vi "ModeMgr.Password Prompt.vi"(9 "Password In":string, 11 "Selected Mode":string) -> (3 "Accepted":bool)   [LabVIEW 2018]
panel:
  in  "Cancel":bool
  out "Action":string
  in  "Password":string
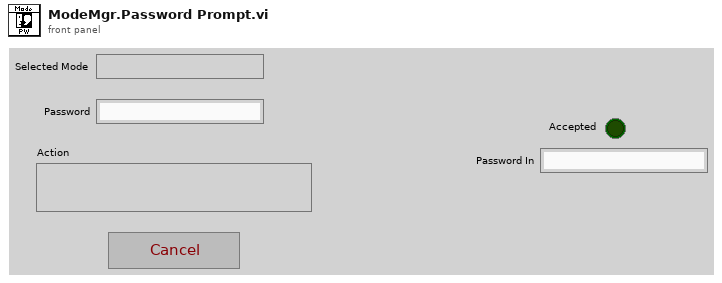
[diagram p1: front panel]
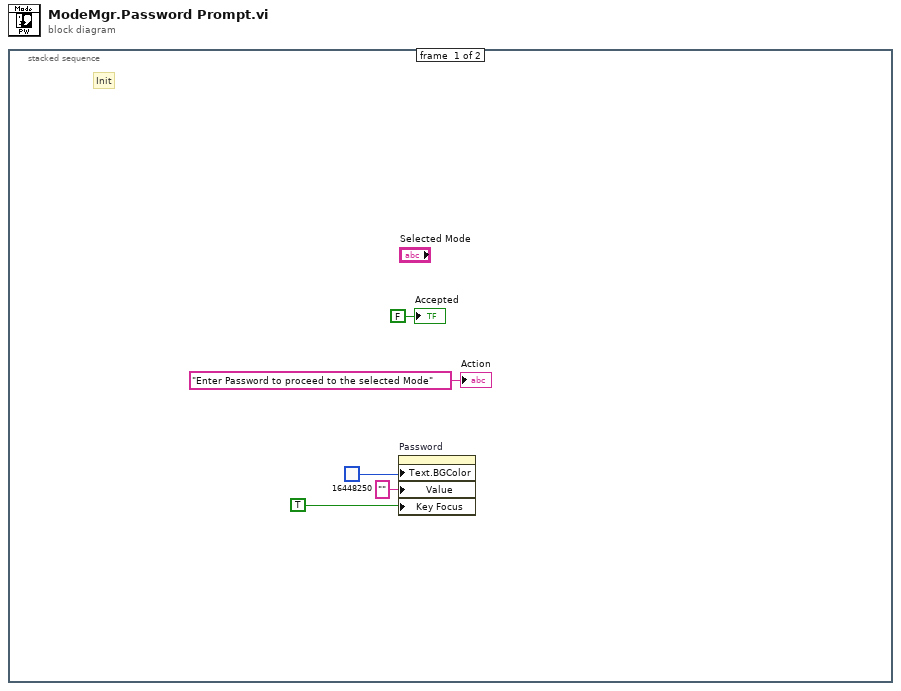
[diagram p0: block diagram]
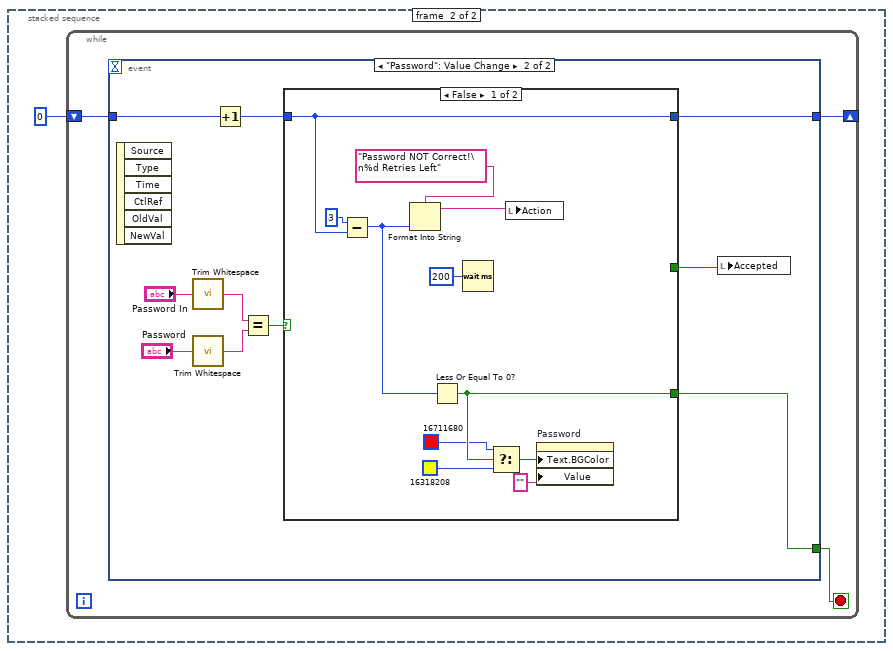
[diagram p2: hidden frame]
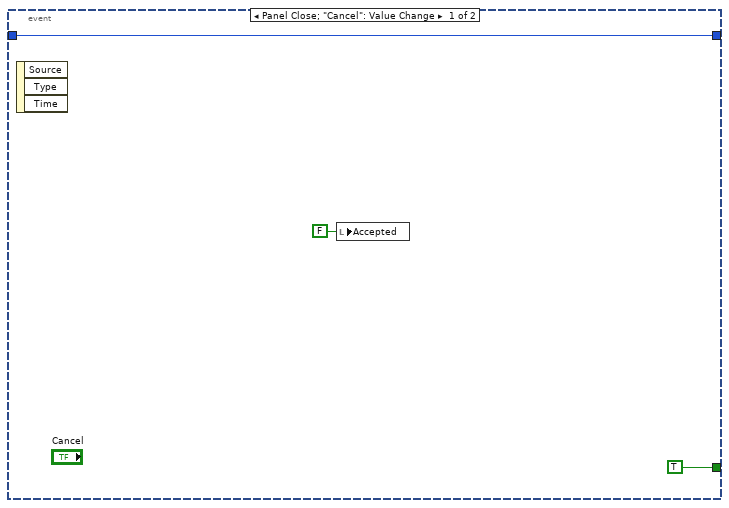
[diagram p3: hidden frame]
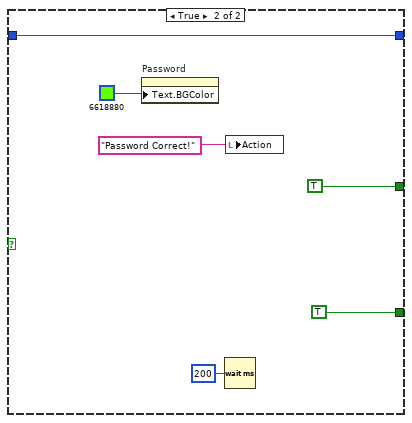
[diagram p4: hidden frame]
diagram:
  n1 = stacked-sequence {
    frame #0 {
      # "Init"
      n2 = property on="Password" class="Str"("Text.BGColor"=u32 16448250, "Value"="" ("Password"), "Key Focus"=TRUE) -> ()  [unwired: 2 in, 2 out]
      "Accepted" <- FALSE ("Accepted")
      "Action" <- "Enter Password to proceed to the selected Mode" ("Action")
    }
    frame #1 {
      n3 = while {
        shift-right: [w7] -> _
        shift-left: 0 -> [w8]
        stop <- w9 stop-if-true
        n4 = event shown="[1] \"Password\": Value Change" {
          selector: _ -> [_ _]
          dyn-events: _ -> [_ _]
          timeout: _ -> [_ _]
          tunnel: [TRUE w16] -> w9
          tunnel: w8 -> [w10 w15]
          tunnel: [w10 w13] -> w7
          event Panel Close; "Cancel": Value Change {
            n5 = event-data() -> ()  [unwired: 1 in, 3 out]
            n6 = local write "Accepted"(FALSE ("Accepted")) -> ()
          }
          event "Password": Value Change {
            n7 = event-data() -> ()  [unwired: 1 in, 6 out]
            n8 = call <vilib>:"Trim Whitespace.vi"("string"="Password In") -> ("trimmed string"=w20:string)  [unwired: 1 in]
            n9 = call <vilib>:"Trim Whitespace.vi"("string"="Password") -> ("trimmed string"=w19:string)  [unwired: 1 in]
            n10 = Increment(x=w15) -> (x+1=w14:i32)
            n11 = Equal?(x=w20, y=w19) -> (x = y?=w18:bool)
            n12 = case shown="False" w18 {
              tunnel: [_ TRUE] -> w17
              tunnel: [w28 TRUE] -> w16
              tunnel: w14 -> [w33 w37]
              tunnel: [w33 w37] -> w13
              frame False {
                n13 = Subtract(x=3, y=w33) -> (x-y=w30:i32)
                n14 = Format Into String(format string="Password NOT Correct!\n%d Retries Left", w30) -> (resulting string=w24:string)  [unwired: 2 in, 1 out]
                n15 = Less Or Equal To 0?(x=w30) -> (x <= 0?=w28:bool)
                n16 = Wait (ms)(milliseconds to wait=u32 200) -> ()  [unwired: 1 out]
                n17 = Select(t=u32 16711680, s=w28, f=u32 16318208) -> (s? t:f=w29:u32)
                n18 = local write "Action"(w24) -> ()
                n19 = property on="Password" class="Str"("Text.BGColor"=w29, "Value"="" ("Password")) -> ()  [unwired: 2 in, 2 out]
              }
              frame True {
                n20 = property on="Password" class="Str"("Text.BGColor"=u32 6618880) -> ()  [unwired: 2 in, 2 out]
                n21 = Wait (ms)(milliseconds to wait=u32 200) -> ()  [unwired: 1 out]
                n22 = local write "Action"("Password Correct!") -> ()
              }
            }
            n23 = local write "Accepted"(w17) -> ()
          }
        }
      }
    }
  }
